vi "test_TCP Protocol Factory.vi"(8 "error in (no error)":errorcluster, 11 "TestCase in":refnum<class "Instrument Addon Scripting API Protocol Factories Unit Tests.lvclass">) -> (0 "error out":errorcluster, 3 "TestCase out":refnum<class "Instrument Addon Scripting API Protocol Factories Unit Tests.lvclass">)   [LabVIEW 2023, in "Instrument Addon Scripting API Protocol Factories Unit Tests.lvclass"]
uses:
  Instrument Addon Scripting API Protocol Factories Unit Tests.lvclass
  <vilib>/addons/_JKI Toolkits/VI Tester/TestCase.llb/TestCase.lvclass
  TCP/TCP.lvclass
  TCP/TCP Settings.ctl
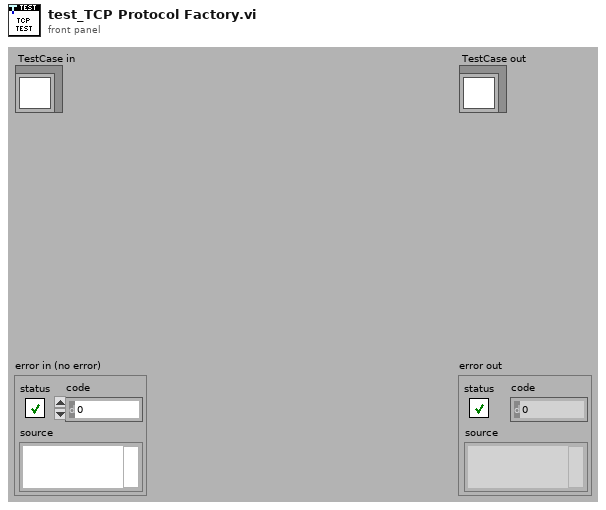
[diagram p1: front panel]
types:
  T1 = typedef "Protocols.lvlib/TCP.lvclass/TCP Settings.ctl" = cluster{"IP Address":string, "Port":u16}
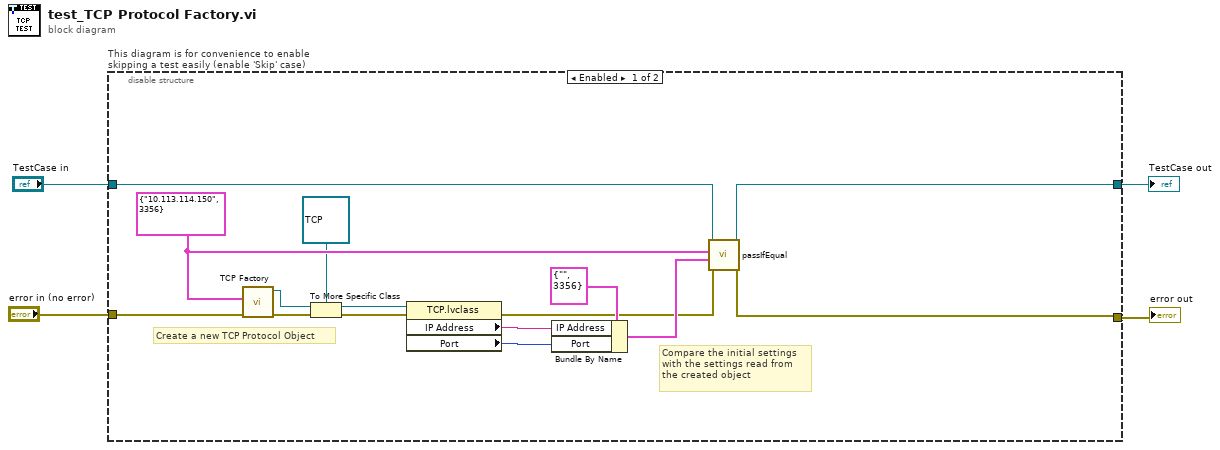
[diagram p0: block diagram]
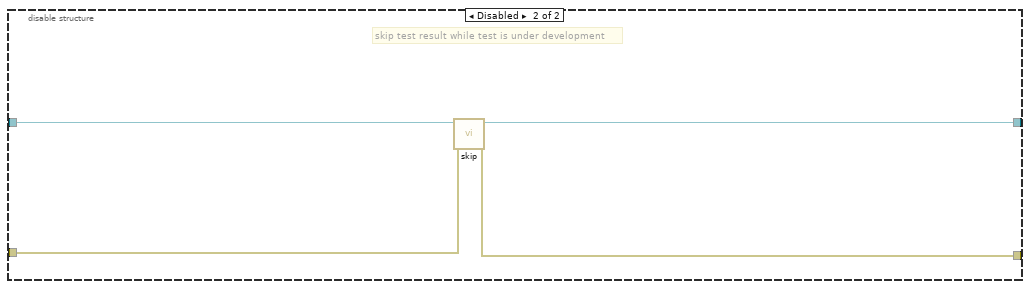
[diagram p2: hidden frame]
diagram:
  n1 = disable-structure "This diagram is for convenience to enable skipping a test easily (enable 'Skip' case)" shown="Enabled" {
    disable-tunnel: "TestCase in" -> [w19 w23]
    disable-tunnel: [w18 w21] -> w1
    disable-tunnel: [w17 w22] -> w3
    disable-tunnel: "error in (no error)" -> [w16 w20]
    frame Enabled {
      w14 = T1 {"IP Address"="10.113.114.150", "Port"=3356} ("TCP Settings")
      # "Compare the initial settings \nwith the settings read from \nthe created object"
      # "Create a new TCP Protocol Object"
      n2 = call "TCP Factory.vi"("error in (no error)"=w16, "TCP settings"=w14) -> ("error out"=w8:errorcluster, "protocol out"=w7:refnum<class "Protocol Parent.lvclass">)  [unwired: 8 in]
      n3 = To More Specific Class(target class=refnum<class "TCP.lvclass"> refnum ("Protocols.lvlib:TCP.lvclass"), reference=w7, error in=w8) -> (specific class reference=w10:refnum<class "TCP.lvclass">, error out=w9:errorcluster)
      n4 = property class="TCP.lvclass"(reference=w10, error in=w9) -> (error out=w5:errorcluster, "IP Address"=w12:string, "Port"=w11:u16)  [unwired: 1 out]
      n5 = Bundle By Name(cluster=T1 {"IP Address"="", "Port"=3356} ("TCP Settings"), "IP Address"=w12, "Port"=w11) -> (w13:T1)
      n6 = call-dynamic "passIfEqual.vi"("error in (no error)"=w5, "y"=w13, "x"=w14, "TestCase in"=w19) -> ("error out"=w17:errorcluster, "TestCase out"=w18:refnum<class "Instrument Addon Scripting API Protocol Factories Unit Tests.lvclass">)  [unwired: 6 in]
    }
    frame Disabled {
      # "skip test result while test is under development"
      n7 = call <vilib>:"skip.vi"("error in (no error)"=w20, "TestCase in"=w23) -> ("error out"=w22:errorcluster, "TestCase out"=w21:refnum<class "Instrument Addon Scripting API Protocol Factories Unit Tests.lvclass">)  [unwired: 8 in]
    }
  }
  "error out" <- w3
  "TestCase out" <- w1
